vi "GetError.vi"(6 "Legacy (f)?":bool, 8 "error in (no error)":errorcluster) -> (0 "error out":errorcluster, 2 "HW Error":errorcluster)   [LabVIEW 2011]
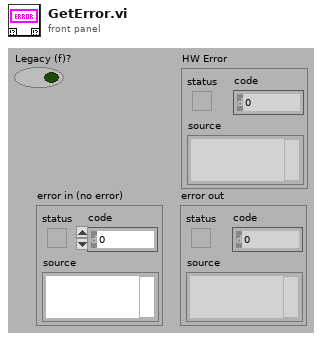
[diagram p1: front panel]
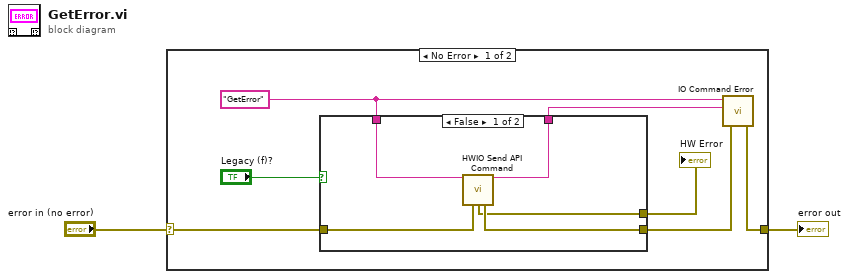
[diagram p0: block diagram]
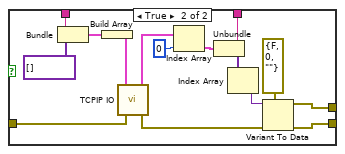
[diagram p2: hidden frame]
diagram:
  n1 = case shown="No Error" "error in (no error)" {
    selector: "error in (no error)" -> [w4 w30]
    tunnel: [w6 w30] -> w2
    frame No Error {
      w9 = "GetError"
      n2 = case shown="False" "Legacy (f)?" {
        tunnel: w9 -> [w14 w27]
        tunnel: [w12 w26] -> w8
        tunnel: [w10 w25] -> w7
        tunnel: [w11 w20] -> w5
        tunnel: w4 -> [w13 w17]
        frame False {
          n3 = call "HWIO Send API Command.vi"("Action"=w14, "error in (no error)"=w13) -> ("Action out"=w11:string, "HWError"=w10:errorcluster, "error out"=w12:errorcluster)  [unwired: 6 in, 5 out]
        }
        frame True {
          n4 = Bundle(w27, "array"=variant[] []) -> (w24:cluster{string, "array":variant[]})  [unwired: 1 out]
          n5 = Build Array(w24) -> (w23:cluster{string, "array":variant[]}[])
          n6 = call "TCPIP IO.vi"("error in (no error)"=w17, "Commands"=w23) -> ("error out"=w28:errorcluster, "Responses"=w22:cluster{string, variant[]}[])  [unwired: 1 in, 3 out]
          n7 = Index Array(array=w22, index=0) -> (element=w21:cluster{string, variant[]})
          n8 = Unbundle(w21) -> (w20:string, w19:variant[])
          n9 = Index Array(array=w19) -> (element=w18:variant)  [unwired: 1 in]
          n10 = Variant To Data(error in=w28, type=errorcluster {"status"=FALSE, "code"=0, "source"=""} ("HW Error"), Variant=w18) -> (data=w25:errorcluster, error out=w26:errorcluster)
        }
      }
      "HW Error" <- w7
      n11 = call "IO Command Error.vi"("error in (no error)"=w8, "Command Returned (\"\")"=w5, "Command Sent (\"\")"=w9) -> ("error out"=w6:errorcluster)  [unwired: 4 out]
    }
    frame Error {
    }
  }
  "error out" <- w2
